vi "ADXL345_Gains.vi"(5 "Y-Axis Gain":dbl, 6 "Z- Axis Gain":dbl, 7 "X-Axis Gain":dbl, 8 "error in":errorcluster, 10 "Raw Accelerometer Data":T4, 11 "Arduino Resource In":T2={"VISA resource"="", "Board Type"=enum."Uno", "Connection Type"=enum."USB / Serial", "Bytes Per Packet (15)"=15}) -> (0 "error out":errorcluster, 2 "Tilt Angles":T1, 3 "Arduino Resource Out":T2={"VISA resource"="", "Board Type"=enum."Uno", "Connection Type"=enum."USB / Serial", "Bytes Per Packet (15)"=15})   [LabVIEW 2012]
uses:
  <vilib>/LabVIEW Interface for Arduino/Type Defs/Arduino Resource.ctl
  <vilib>/LabVIEW Interface for Arduino/Type Defs/Board Type.ctl
  <vilib>/LabVIEW Interface for Arduino/LabVIEW Interface for Arduino.lvlib
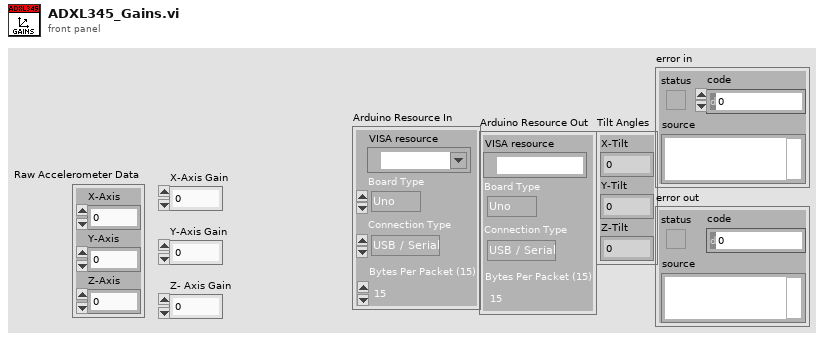
[diagram p1: front panel]
types:
  T1 = cluster{"X-Tilt":dbl, "Y-Tilt":dbl, "Z-Tilt":dbl}
  T2 = typedef "LabVIEW Interface for Arduino.lvlib/Arduino Resource.ctl" = cluster{"VISA resource":refnum<visa-resource-name>, "Board Type":T3, "Connection Type":enum8{"USB / Serial"}, "Bytes Per Packet (15)":u8}
  T3 = typedef "LabVIEW Interface for Arduino.lvlib/Board Type.ctl" = enum16{"Uno", "Dimuelanove w/Atmega 328", "Mega 2560"}
  T4 = cluster{"X-Axis":i32, "Y-Axis":i32, "Z-Axis":i32}
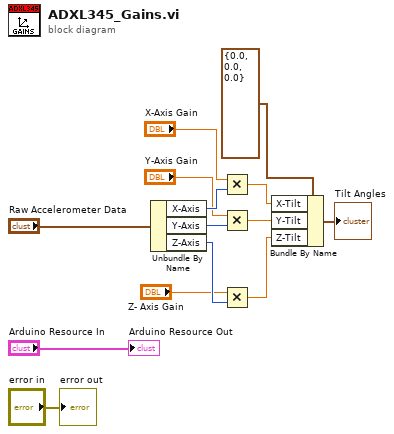
[diagram p0: block diagram]
diagram:
  n1 = Unbundle By Name("Raw Accelerometer Data") -> ("X-Axis"=w12:i32, "Y-Axis"=w13:i32, "Z-Axis"=w14:i32)
  n2 = Multiply(x="X-Axis Gain", y=w12) -> (x*y=w5:dbl)
  n3 = Multiply(x="Y-Axis Gain", y=w13) -> (x*y=w4:dbl)
  n4 = Multiply(x="Z- Axis Gain", y=w14) -> (x*y=w3:dbl)
  n5 = Bundle By Name(cluster=T1 {"X-Tilt"=0.0, "Y-Tilt"=0.0, "Z-Tilt"=0.0} ("input cluster"), "X-Tilt"=w5, "Y-Tilt"=w4, "Z-Tilt"=w3) -> (→"Tilt Angles":T1)
  "Arduino Resource Out" <- "Arduino Resource In"
  "error out" <- "error in"
